vi "myXi_UpdateTrigger.vi"(8 "error in (no error)":errorcluster, 9 "trigger":bool, 11 "xiCam IN":refnum<k24>) -> (0 "error out":errorcluster, 3 "xiCam Out":refnum<k24>)   [LabVIEW 2018]
uses:
  C:/XIMEA/API/x64/xiApi.NETX64.dll
  VisionLibrariesXimea/xiLib/xiLIB_64bit/xiLIB/xiCamLib/xiCam/PRM/PRM/PRM_v2.ctl
  VisionLibrariesXimea/xiLib/xiLIB_64bit/xiLIB/xiCamLib/xiCam/PRM/TRG_SOURCE/TRG_SOURCE.ctl
  VisionLibrariesXimea/xiLib/xiLIB_64bit/xiLIB/xiCamLib/xiCam/PRM/GPI_MODE/GPI_MODE.ctl
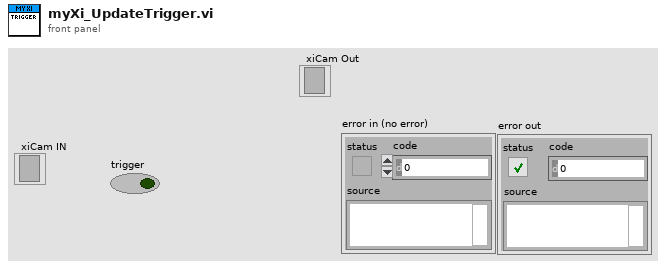
[diagram p1: front panel]
types:
  T1 = typedef "PRM_v2.ctl" = enum16{"ACQ_BUFFER_SIZE", "ACQ_FRAME_BURST_COUNT", "ACQ_TIMING_MODE", "ACQ_TRANSPORT_BUFFER_SIZE", "AE_MAX_LIMIT", "AEAG", "AEAG_LEVEL", "API_VERSION", "AG_MAX_LIMIT", "APPLY_CMS", "AUTO_BANDWIDTH_CALCULATION", "AUTO_WB", "AVAILABLE_BANDWIDTH", "AVAILABLE_BANDWIDTH_MAX", "AVAILABLE_BANDWIDTH_MIN", "BPC", "BUFFER_POLICY", "BUFFERS_QUEUE_SIZE", "CC_MATRIX_00", "CC_MATRIX_01", "CC_MATRIX_02", "CC_MATRIX_03", "CC_MATRIX_10", "CC_MATRIX_11", "CC_MATRIX_12", "CC_MATRIX_13", "CC_MATRIX_20", "CC_MATRIX_21", "CC_MATRIX_22", "CC_MATRIX_23", "CC_MATRIX_30", "CC_MATRIX_31", "CC_MATRIX_32", "CC_MATRIX_33", "CHIP_TEMP", "CMS", "COLOR_FILTER_ARRAY", "COOLING", "DEBOUNCE_EN", "DEBOUNCE_POL", "DEBOUNCE_T0", "DEBOUNCE_T1", "DEBUG_LEVEL", "DEFAULT_CC_MATRIX", "DEVICE_INSTANCE_PATH", "DEVICE_MODEL_ID", "DEVICE_NAME", "DEVICE_SN", "DEVICE_TYPE", "DEVICE_USER_ID", "DOWNSAMPLING", "DOWNSAMPLING_MAX", "DOWNSAMPLING_MIN", "DOWNSAMPLING_TYPE", "DRV_VERSION", "EXP_PRIORITY", "EXPOSURE", "EXPOSURE_DIRECT_UPDATE", "EXPOSURE_MAX", "EXPOSURE_MIN", "FFS_FILE_NAME", "FPGA1_VERSION", "FRAMERATE", "FRAMERATE_MAX", "FRAMERATE_MIN", "FREE_FFS_SIZE", "GAIN", "GAIN_DIRECT_UPDATE", "GAIN_MAX", "GAIN_MIN", "GAMMAC", "GAMMAY", "GPI_LEVEL", "GPI_MODE", "GPI_SELECTOR", "GPI_SELECTOR_MAX", "GPI_SELECTOR_MIN", "GPO_MODE", "GPO_SELECTOR", "GPO_SELECTOR_MAX", "GPO_SELECTOR_MIN", "HDR", "HDR_T1", "HDR_T2", "HEIGHT", "HEIGHT_MAX", "HEIGHT_MIN", "HOUSE_TEMP", "IMAGE_DATA_FORMAT", "IMAGE_IS_COLOR", "INPUT_CMS_PROFILE", "IS_COOLED", "IS_DEVICE_EXIST", "KNEEPOINT1", "KNEEPOINT2", "LED_MODE", "LED_SELECTOR", "LED_SELECTOR_MAX", "LED_SELECTOR_MIN", "LIMIT_BANDWIDTH", "LIMIT_BANDWIDTH_MAX", "LIMIT_BANDWIDTH_MIN", "LUT_EN", "LUT_INDEX", "LUT_INDEX_MAX", "LUT_INDEX_MIN", "LUT_VALUE", "LUT_VALUE_MAX", "LUT_VALUE_MIN", "MANUAL_WB", "MCU1_VERSION", "MCU2_VERSION", "OFFSET_X", "OFFSET_X_MAX", "OFFSET_X_MIN", "OFFSET_Y", "OFFSET_Y_MAX", "OFFSET_Y_MIN", "OUTPUT_CMS_PROFILE", "OUTPUT_DATA_BIT_DEPTH", "OUTPUT_DATA_PACKING", "READ_FILE_FFS", "RECENT_FRAME", "SENSOR_DATA_BIT_DEPTH", "SENSOR_MODE", "SENSOR_TAPS", "SHARPNESS", "SHUTTER_TYPE", "TARGET_TEMP", "TRG_DELAY", "TRG_SELECTOR", "TRG_SOFTWARE", "TRG_SOURCE", "USED_FFS_SIZE", "WB_KB", "WB_KG", "WB_KR", "WIDTH", "WIDTH_MAX", "WIDTH_MIN", "WRITE_FILE_FFS", "ACQ_BUFFER_SIZE_UNIT", "ACQ_TRANSPORT_BUFFER_COMMIT", "AEAG_ROI_HEIGHT", "AEAG_ROI_OFFSET_X", "AEAG_ROU_OFFSET_Y", "AEAG_ROI_WIDTH", "API_CONTEXT_LIST", "BINNING_HORIZONTAL", "BINNING_SELECTOR", "BINNING_VERTICAL", "COLUMN_FPN_CORRECTION", "COUNTER_SELECTOR", "COUNTER_VALUE", "DECIMATION_HORIZONTAL", "DECIMATION_SELECTOR", "DECIMATION_VERTICAL", "DEVICE_ID", "DEVICE_LOCATION_PATH", "DEVICE_MANIFEST", "DEVICE_RESET", "DEVICE_SENS_SN", "EXPOSURE_BURST_COUNT", "FFS_ACCESS_KEY", "GAIN_SELECTOR", "HW_REVISION", "IMAGE_BLACK_LEVEL", "IMAGE_DATA_BIT_DEPTH", "IMAGE_DATA_FORMAT_RGB32_ALPHA", "IMAGE_PAYLOAD_SIZE", "LENS_APERTURE_VALUE", "LENS_FEATURE", "LENS_FEATURE_SELECTOR", "LENS_FOCAL_LENGTH", "LENS_FOCUS_DISTANCE", "LENS_FOCUS_MOVE", "LENS_FOCUS_MOVEMENT_VALUE", "LENS_MODE", "OUTPUT_DATA_PACKING_TYPE", "SENSOR_CLOCK_FREQ_HZ", "SENSOR_CLOCK_FREQ_INDEX", "SENSOR_FEATURE_SELECTOR", "SENSOR_FEATURE_VALUE", "SENSOR_OUTPUT_CHANNEL_COUNT", "TRANSPORT_PIXEL_FORMAT", "TS_RST_MODE", "TS_RST_SOURCE"}
  T2 = typedef "GPI_MODE.ctl" = enum16{"OFF", "TRIGGER", "EXT_EVENT"}
  T3 = typedef "TRG_SOURCE.ctl" = enum16{"OFF", "EDGE_RISING", "EDGE_FALLING", "SOFTWARE"}
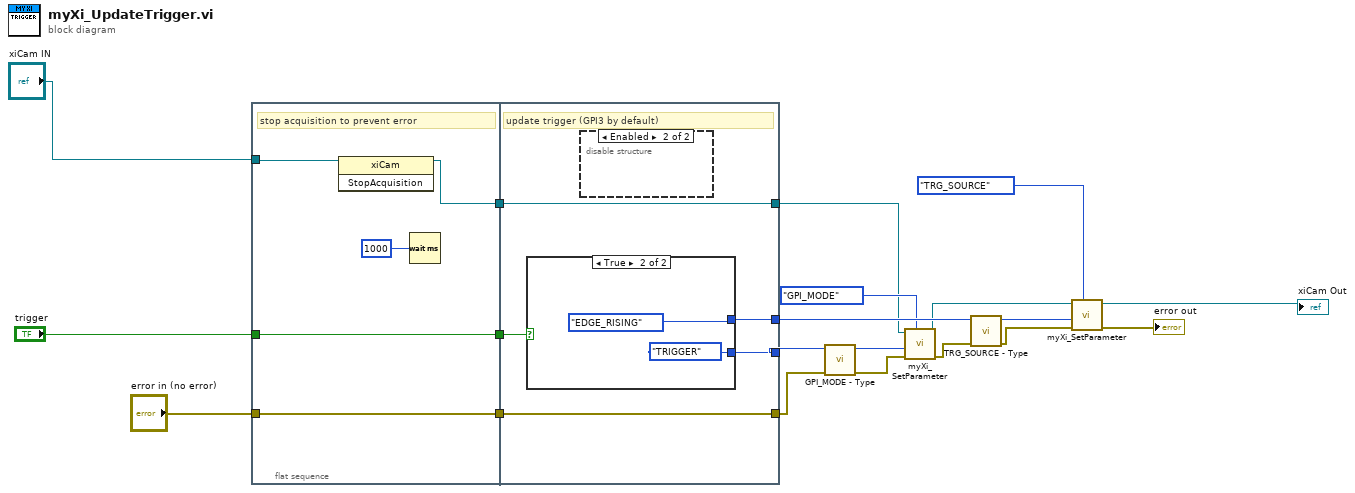
[diagram p0: block diagram]
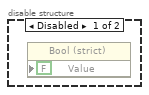
[diagram p2: hidden frame]
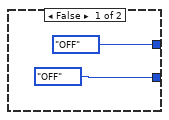
[diagram p3: hidden frame]
diagram:
  n1 = flat-sequence {
    tunnel: "trigger" -> [w25]
    tunnel: [w25] -> w8
    tunnel: "error in (no error)" -> [w24]
    tunnel: [w24] -> w5
    tunnel: "xiCam IN" -> [w23]
    tunnel: [w22] -> w3
    tunnel: [w30] -> w17
    tunnel: [w28] -> w13
    tunnel: w8 -> [w29]
    tunnel: [w27] -> w6
    tunnel: w5 -> [w27]
    tunnel: [w26] -> w2
    tunnel: w3 -> [w26]
    frame #0 {
      # "stop acquisition to prevent error"
      n2 = invoke class="xiCam" method="StopAcquisition"(reference=w23) -> (reference out=w22:refnum<k24>)  [unwired: 2 in, 2 out]
      n3 = Wait (ms)(milliseconds to wait=u32 1000) -> ()  [unwired: 1 out]
    }
    frame #1 {
      # "update trigger (GPI3 by default)"
      n4 = case shown="True" w29 {
        tunnel: [TRG_SOURCE."OFF" ("TRG_SOURCE") TRG_SOURCE."EDGE_RISING" ("TRG_SOURCE")] -> w30
        tunnel: [GPI_MODE."OFF" ("GPI_MODE") GPI_MODE."TRIGGER" ("GPI_MODE")] -> w28
        frame False {
        }
        frame True {
        }
      }
      n5 = disable-structure shown="Enabled" {
        frame Disabled {
          n6 = property on="Property Node" class="Bool (strict)"("Value"=FALSE ("Play Button")) -> ()  [unwired: 2 in, 2 out]
        }
        frame Enabled {
        }
      }
    }
  }
  n7 = call "GPI_MODE - Type.vi"("error in (no error)"=w6, "GPI_MODE"=w13) -> ("error out"=w11:errorcluster, "GPI_MODE_VALUE"=w12:i32)  [unwired: 8 in]
  n8 = call "myXi_SetParameter.vi"("input PRM"=PRM_v2."GPI_MODE", "error in"=w11, "input value I32"=w12, "xiCam IN"=w2) -> ("error out"=w16:errorcluster, "xiCam Out"=w15:refnum<k24>)  [unwired: 6 in]
  n9 = call "TRG_SOURCE - Type.vi"("error in (no error)"=w16, "TRG_SOURCE"=w17) -> ("error out"=w18:errorcluster, "TRG_SOURCE_VALUE"=w19:i32)  [unwired: 8 in]
  n10 = call "myXi_SetParameter.vi"("input PRM"=PRM_v2."TRG_SOURCE", "error in"=w18, "input value I32"=w19, "xiCam IN"=w15) -> ("error out"=→"error out":errorcluster, "xiCam Out"=→"xiCam Out":refnum<k24>)  [unwired: 6 in]
